vi "Change Precision Type.vi"(8 "error in (no error)":errorcluster, 10 "Precision Type":T1, 11 "Numeric Data Type in":refnum<class "Numeric Data Type.lvclass">) -> (0 "error out":errorcluster, 3 "Numeric Data Type out":refnum<class "Numeric Data Type.lvclass">)   [LabVIEW 2018, in "Numeric Data Type.lvclass"]
uses:
  Numeric Data Type.lvclass
  Precision Type.ctl
  Numeric Data Type.lvclass/Numeric Data Type.ctl
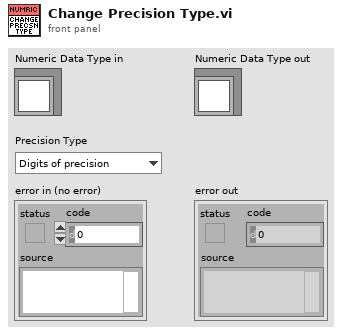
[diagram p1: front panel]
types:
  T1 = typedef "Numeric Data Type.lvclass/Precision Type.ctl" = enum16{"Digits of precision", "Significant digits"}
  T2 = typedef "Numeric Data Type.lvclass/Numeric Info.ctl" = cluster{"Minimum Field Width":i32, "Digits of Precision":i32, "Numeric Format":T3, "Precision Type":T1, "Hide trailing zeros":bool, "exponent":bool, "just/pad":T4, "Modifiers":string}
  T3 = typedef "Numeric Data Type.lvclass/Numeric Format Enum.ctl" = enum16{"Floating Point Notation", "Scientific Notation", "Engineering Notation", "SI Notation", "<not used>", "Decimal", "Hexadecimal", "Octal", "Binary", "<not used 2>", "Absolute Time", "Relative Time"}
  T4 = typedef "Numeric Data Type.lvclass/Padding.ctl" = enum16{"Pad with spaces on left", "Pad with spaces on right", "Pad with zeros on left"}
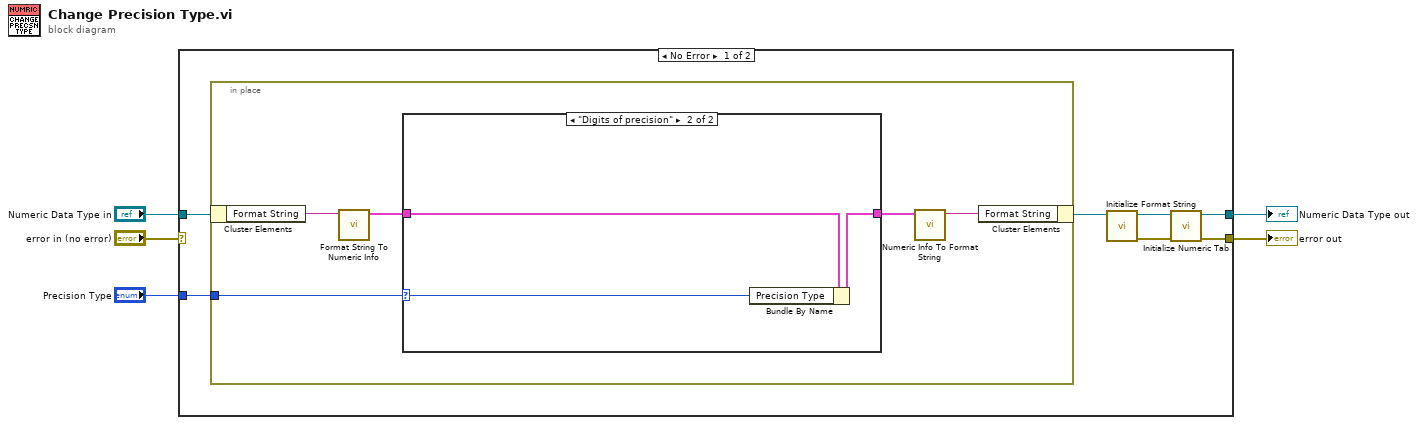
[diagram p0: block diagram]
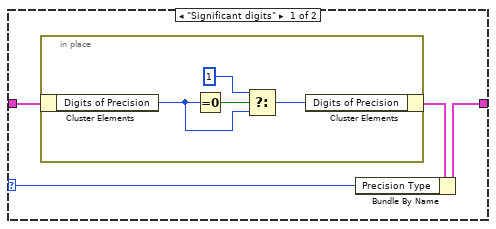
[diagram p2: hidden frame]
diagram:
  n1 = case shown="No Error" "error in (no error)" {
    selector: "error in (no error)" -> [_ w30]
    tunnel: [w6 w30] -> w4
    tunnel: [w8 w29] -> w2
    tunnel: "Numeric Data Type in" -> [w12 w29]
    tunnel: "Precision Type" -> [w10 _]
    frame No Error {
      n2 = in-place {
        in-place-border: w10 -> [w13]
        n3 = in-place-cluster #1(w12) -> ("Format String"=w17:string)
        n4 = call "Format String To Numeric Info.vi"("Format String"=w17) -> ("Numeric Format & Precision Info"=w16:T2)  [unwired: 10 in]
        n5 = case shown="\"Digits of precision\"" w13 {
          selector: w13 -> [w20 w27]
          tunnel: w16 -> [w19 w26]
          tunnel: [w21 w28] -> w15
          frame "Significant digits" {
            n6 = in-place {
              n7 = in-place-cluster #2(w19) -> ("Digits of Precision"=w24:i32)
              n8 = Equal To 0?(x=w24) -> (x = 0?=w25:bool)
              n9 = Select(t=1, s=w25, f=w24) -> (s? t:f=w23:i32)
              n10 = in-place-cluster #2("Digits of Precision"=w23) -> (w18:T2)
            }
            n11 = Bundle By Name(cluster=w18, "Precision Type"=w20) -> (w21:T2)
          }
          frame "Digits of precision" {
            n12 = Bundle By Name(cluster=w26, "Precision Type"=w27) -> (w28:T2)
          }
        }
        n13 = call "Numeric Info To Format String.vi"("Numeric Format & Precision Info"=w15) -> ("Format String"=w14:string)  [unwired: 10 in]
        n14 = in-place-cluster #1("Format String"=w14) -> (w11:refnum<class "Numeric Data Type.lvclass">)
      }
      n15 = call "Initialize Format String.vi"("Numeric Data Type in"=w11) -> ("error out"=w7:errorcluster, "Numeric Data Type (dup)"=w9:refnum<class "Numeric Data Type.lvclass">)  [unwired: 9 in]
      n16 = call "Initialize Numeric Tab.vi"("error in (no error)"=w7, "Numeric Data Type in"=w9) -> ("error out"=w6:errorcluster, "Numeric Data Type (dub)"=w8:refnum<class "Numeric Data Type.lvclass">)  [unwired: 8 in]
    }
    frame Error {
    }
  }
  "error out" <- w4
  "Numeric Data Type out" <- w2
